vi "Unsubscribe.vi"(8 "error in (no error)":errorcluster, 10 "SubscriptionPolicy":T1, 11 "IObserver in":refnum<class "IObserver.lvclass">) -> (0 "error out":errorcluster, 3 "IObserver out":refnum<class "IObserver.lvclass">)   [LabVIEW 2015, in "IObserver.lvlib" / "IObserver.lvclass"]
doc: "<License>\nCopyright © 2017 Composed Systems, LLC | All rights reserved\nwww.composed.io\n\nAuthor: Ethan Stern <ethan.stern@composed.io>\n\nThis software is provided \"AS IS\" WITHOUT WARRANTIES, either express or implied, AND IS FOR EDUCATIONAL PURPOSES ONLY.\n</License>"
uses:
  IObserver.lvclass
  IMediator/ISubscriptionPolicy/ISubscriptionPolicy Reference.ctl
  IMediator/ISubscriptionPolicy/ISubscriptionPolicy.lvclass
  IObserver.lvclass/IObserver.ctl
  AbstractMessages/PreAddressedMsg/PreAddressedMsg.lvclass/PreAddressedMsg.ctl
  IMediator/IMediator Messages/Unsubscribe Msg/Unsubscribe Msg.lvclass/Unsubscribe Msg.ctl
  <vilib>/ActorFramework/Message Enqueuer/Message Enqueuer.lvclass/Message Enqueuer.ctl
  <vilib>/ActorFramework/Message Enqueuer/Enqueue.vi
  AbstractMessages/PreAddressedMsg/Read Return Address.vi
  <vilib>/ActorFramework/Message Priority Queue/Priority Enqueue.vi
  IMediator/IMediator Messages/Unsubscribe Msg/Unsubscribe Msg.lvclass
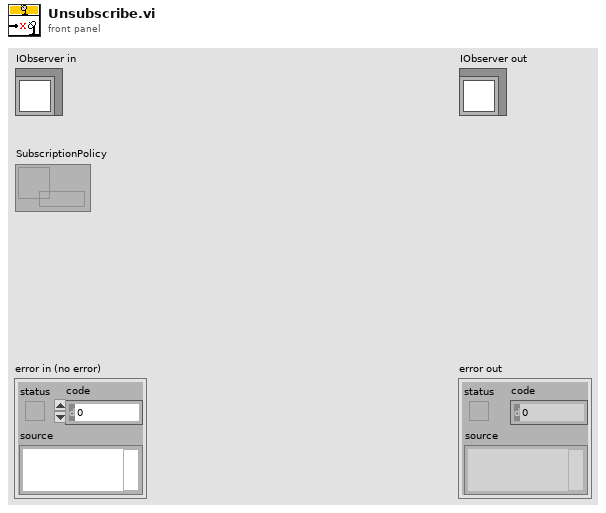
[diagram p1: front panel]
types:
  T1 = typedef "IMediator.lvlib/ISubscriptionPolicy.lvclass/ISubscriptionPolicy Reference.ctl" = refnum<data-value>
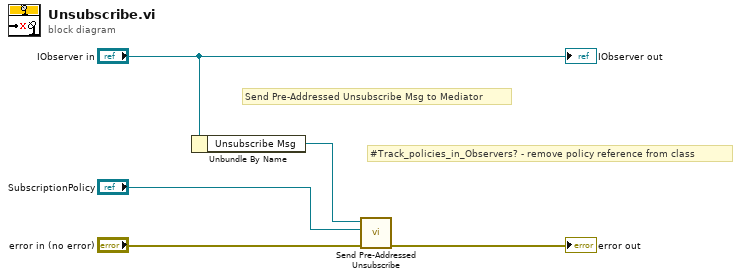
[diagram p0: block diagram]
diagram:
  # "#Track_policies_in_Observers? - remove policy reference from class"
  # "Send Pre-Addressed Unsubscribe Msg to Mediator"
  n1 = Unbundle By Name("IObserver in") -> ("Unsubscribe Msg"=w4:refnum<class "Unsubscribe Msg.lvclass">)
  n2 = call "Send Pre-Addressed Unsubscribe.vi"("error in (no error)"="error in (no error)", "SubscriptionPolicy"="SubscriptionPolicy", "Unsubscribe Msg In"=w4) -> ("error out"=→"error out":errorcluster)  [unwired: 8 in]
  "IObserver out" <- "IObserver in"
